vi "AssembleBLMultiplotScript-Spectra.vi"(0 "gnuplotIn":string, 1 "Title":string="PSD of longitudinal velocity", 5 "SpectrumFilename":string="spec.dat", 9 "f.E(f) Bounds":T1={"Min"={"Auto"=FALSE, "Value"=5.0}, "Max"={"Auto"=FALSE, "Value"=2000.0}}, 12 "f Bounds":T1={"Min"={"Auto"=FALSE, "Value"=0.0}, "Max"={"Auto"=FALSE, "Value"=1.2}}) -> (4 "gnuplotOut":string)   [LabVIEW 2013]
uses:
  minAndMax.ctl
  AutoManualNumber.ctl
  axisName.ctl
  ticsAndGrids.ctl
  tics.ctl
  grids.ctl
  legendProperties.ctl
  legendAppearance.ctl
  alignment.ctl
  at.ctl
panel:
  out "SpectrumSection":string
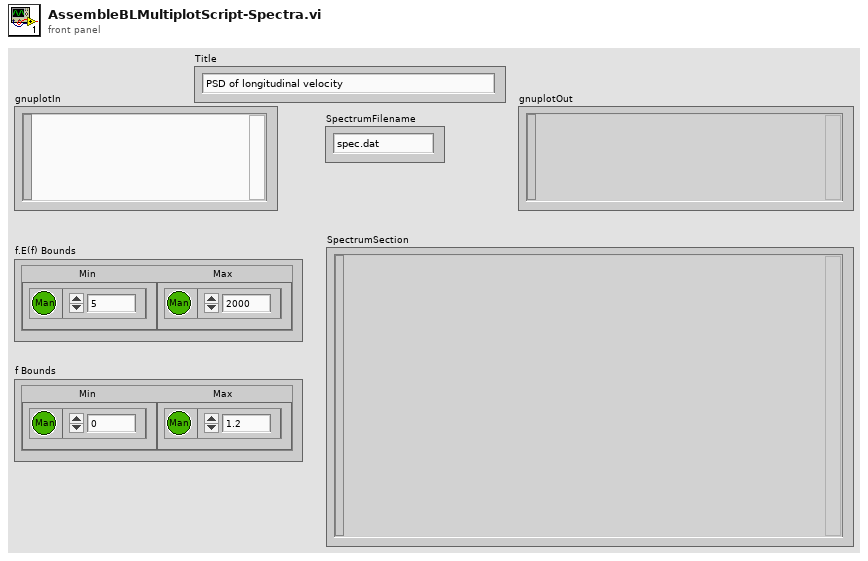
[diagram p1: front panel]
types:
  T1 = typedef "minAndMax.ctl" = cluster{"Min":T2, "Max":T2}
  T2 = typedef "AutoManualNumber.ctl" = cluster{"Auto":bool, "Value":dbl}
  T3 = typedef "axisName.ctl" = string
  T4 = typedef "legendProperties.ctl" = cluster{"Appearance":T5, "Alignment":T6, "Location":string, "\"At\" location":T7}
  T5 = typedef "legendAppearance.ctl" = cluster{"layout":string, "text-sample order":string, "key order":string, "surroundingBox":string}
  T6 = typedef "alignment.ctl" = cluster{"Horizontal":string, "Vertical":string}
  T7 = typedef "at.ctl" = cluster{"XcoordSys":string, "YcoordSys":string, "Xvalue":dbl, "Yvalue":dbl}
  T8 = typedef "ticsAndGrids.ctl" = cluster{"tics":T9, "Grids":T10, "Mapping":enum8{"Lin", "Log"}}
  T9 = typedef "tics.ctl" = cluster{"ticMin":dbl, "ticStep":dbl, "ticMax":dbl, "minorDivsPerMajor":i32, "ticSpacing":enum16{"Auto Tics", "Fixed spacing", "Fixed Minimum and Spacing", "Start, Spacing and Maximum", "Approx n Tics (rounded)"}, "ticPosition":enum16{"Inside, no mirror", "Inside, mirrored", "Outside, no mirror", "Outside, mirrored", "Invisible"}}
  T10 = typedef "grids.ctl" = cluster{"Gridlines":enum16{"No grids", "Major grid", "Minor grid", "Major and Minor"}, "Zeroaxis":enum16{"No zero axis", "Show zero axis"}}
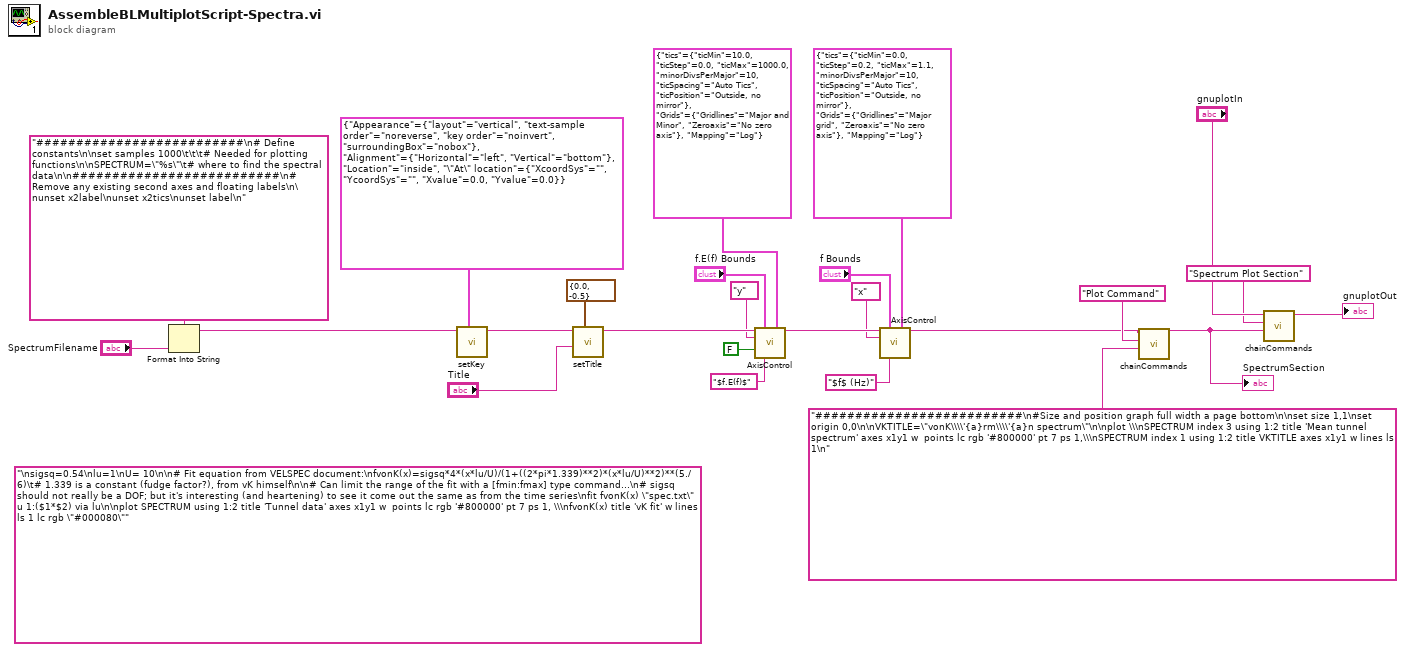
[diagram p0: block diagram]
diagram:
  (unwired) "\nsigsq=0.54\nlu=1\nU= 10\n\n# Fit equation from VELSPEC document:\nfvonK(x)=sigsq*4*(x*lu/U)/(1+((2*pi*1.339)**2)*(x*lu/U)**2)**(5./6)\t# 1.339 is a constant (fudge factor?), from vK himself\n\n# Can limit the range of the fit with a [fmin:fmax] type command...\n# sigsq should not really be a DOF; but it's interesting (and heartening) to see it come out the same as from the time series\nfit fvonK(x) \"spec.txt\" u 1:($1*$2) via lu\n\nplot SPECTRUM using 1:2 title 'Tunnel data' axes x1y1 w  points lc rgb '#800000' pt 7 ps 1, \\\nfvonK(x) title 'vK fit' w lines ls 1 lc rgb \"#000080\""
  n1 = Format Into String(format string="##########################\n# Define constants\n\nset samples 1000\t\t\t# Needed for plotting functions\n\nSPECTRUM=\"%s\"\t# where to find the spectral data\n\n##########################\n# Remove any existing second axes and floating labels\n\nunset x2label\nunset x2tics\nunset label\n" ("Command"), "SpectrumFilename") -> (resulting string=w5:string)  [unwired: 2 in, 1 out]
  n2 = call "setKey.vi"("LegendProperties"=T4 {"Appearance"={"layout"="vertical", "text-sample order"="noreverse", "key order"="noinvert", "surroundingBox"="nobox"}, "Alignment"={"Horizontal"="left", "Vertical"="bottom"}, "Location"="inside", "\"At\" location"={"XcoordSys"="", "YcoordSys"="", "Xvalue"=0.0, "Yvalue"=0.0}}, "String in"=w5) -> ("String out"=w25:string)  [unwired: 8 in, 1 out]
  n3 = call "setTitle.vi"("Offset"=cluster{"horizontal":dbl, "vertical":dbl} {"horizontal"=0.0, "vertical"=-0.5}, "Title"="Title", "String in"=w25) -> ("String out"=w24:string)  [unwired: 7 in, 1 out]
  n4 = call "AxisControl.vi"("String in"=w24, "AxisBounds"="f.E(f) Bounds", "ticsAndGrids"=T8 {"tics"={"ticMin"=10.0, "ticStep"=0.0, "ticMax"=1000.0, "minorDivsPerMajor"=10, "ticSpacing"=enum."Auto Tics", "ticPosition"=enum."Outside, no mirror"}, "Grids"={"Gridlines"=enum."Major and Minor", "Zeroaxis"=enum."No zero axis"}, "Mapping"=enum."Log"}, "Axis"=T3 "y", "ShowNumbers?"=FALSE, "Axis Label"="$f.E(f)$") -> ("String out"=w20:string)  [unwired: 8 in, 1 out]
  n5 = call "AxisControl.vi"("String in"=w20, "AxisBounds"="f Bounds", "ticsAndGrids"=T8 {"tics"={"ticMin"=0.0, "ticStep"=0.2, "ticMax"=1.1, "minorDivsPerMajor"=10, "ticSpacing"=enum."Auto Tics", "ticPosition"=enum."Outside, no mirror"}, "Grids"={"Gridlines"=enum."Major grid", "Zeroaxis"=enum."No zero axis"}, "Mapping"=enum."Log"}, "Axis"=T3 "x", "Axis Label"="$f$ (Hz)") -> ("String out"=w10:string)  [unwired: 9 in, 1 out]
  n6 = call "chainCommands.vi"("Command"="##########################\n#Size and position graph full width a page bottom\n\nset size 1,1\nset origin 0,0\n\nVKTITLE=\"vonK\\\\'{a}rm\\\\'{a}n spectrum\"\n\nplot \\\nSPECTRUM index 3 using 1:2 title 'Mean tunnel spectrum' axes x1y1 w  points lc rgb '#800000' pt 7 ps 1,\\\nSPECTRUM index 1 using 1:2 title VKTITLE axes x1y1 w lines ls 1\n", "Comments"="Plot Command", "StringIn"=w10) -> ("StringOut"=w4:string)  [unwired: 8 in]
  "SpectrumSection" <- w4
  n7 = call "chainCommands.vi"("Command"=w4, "Comments"="Spectrum Plot Section", "StringIn"="gnuplotIn") -> ("StringOut"=→"gnuplotOut":string)  [unwired: 8 in]
